vi "ROS_MasterSaveHTML.vi"(3 "Latest Request":string, 5 "Current":T3) -> ()   [LabVIEW 2015]
doc: "saves HTML file for Master"
uses:
  ROS_Master.ctl
  ROS_Topic.ctl
  ROS_Node.ctl
  ROS_Service.ctl
  SubVIs/_ROSControl.ctl
  SubVIs/_ROSDirection.ctl
panel:
  in  "ROS":T1={"topic port"=0, "Node"="", "topic"="", "type"="", "node port"=0, "error "={"status"=FALSE, "code"=0, "source"=""}, "Direction"=enum."Node", "Update (ms)"=1, "FIFO size"=1}
  out "HTML":string
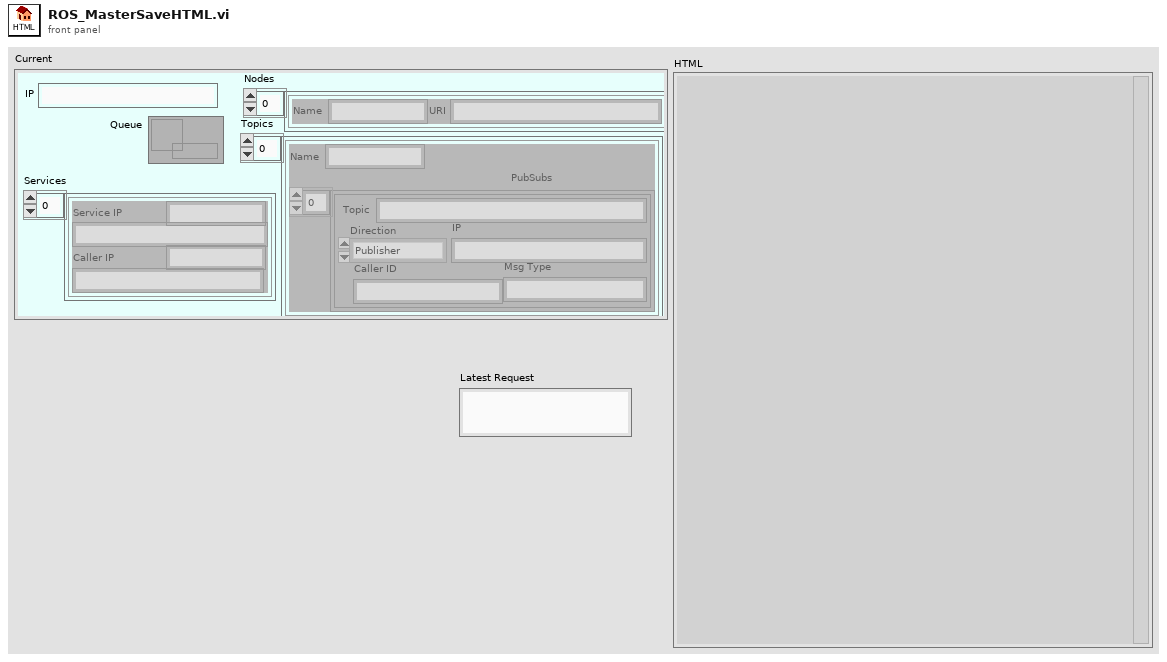
[diagram p1: front panel]
types:
  T1 = typedef "_ROSControl.ctl" = cluster{"topic port":u16, "Node":string, "topic":string, "type":string, "node port":u16, "error ":errorcluster, "Direction":T2, "Update (ms)":u16, "FIFO size":u16}
  T2 = typedef "_ROSDirection.ctl" = enum16{"Node", "Publisher", "Subscriber", "ServiceClient", "ServiceProvider"}
  T3 = typedef "ROS_Master.ctl" = cluster{"IP":string, "Topics":cluster{"Name":string, "PubSubs":T4[]}[], "Nodes":T5[], "Services":T6[], "Queue":refnum<queue>}
  T4 = typedef "ROS_Topic.ctl" = cluster{"Caller ID":string, "IP":string, "Msg Type":string, "Direction":enum16{"Publisher", "Subscriber"}, "Topic":string}
  T5 = typedef "ROS_Node.ctl" = cluster{"Name":string, "URI":string}
  T6 = typedef "ROS_Service.ctl" = cluster{"Service":string, "Service IP":string, "Caller IP":string, "Caller ID":string}
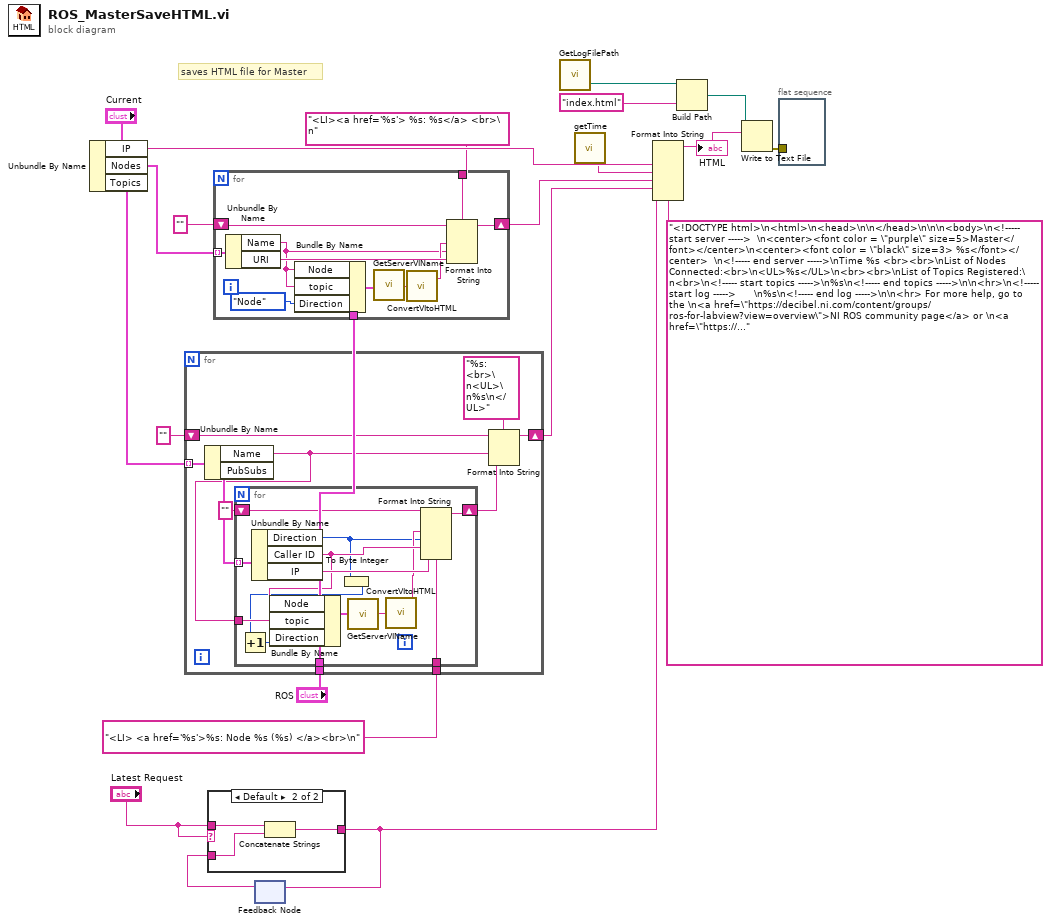
[diagram p0: block diagram]
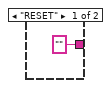
[diagram p2: hidden frame]
diagram:
  # "saves HTML file for Master"
  n1 = Unbundle By Name("Current") -> ("IP"=w19:string, "Nodes"=w18:T5[], "Topics"=w14:cluster{"Name":string, "PubSubs":T4[]}[])
  n2 = for {
    tunnel: w14 -> [w31] mode=indexing
    shift-right: [w29] -> w13
    shift-left: "" -> [w28]
    tunnel: "ROS" -> [w24]
    tunnel: "<LI> <a href='%s'>%s: Node %s (%s) </a><br>\n" ("format string") -> [w23]
    n3 = Unbundle By Name(w31) -> ("Name"=w22:string, "PubSubs"=w27:T4[])
    n4 = for {
      tunnel: w27 -> [w45] mode=indexing
      shift-right: [w42] -> w25
      shift-left: "" -> [w43]
      tunnel: w24 -> [w39]
      tunnel: w22 -> [w37]
      tunnel: w23 -> [w36]
      n5 = Unbundle By Name(w45) -> ("Direction"=w34:enum16{"Publisher", "Subscriber"}, "Caller ID"=w38:string, "IP"=w44:string)
      n6 = To Byte Integer(number=w34) -> (8bit integer=w32:i8)
      n7 = Increment(x=w32) -> (x+1=w33:i8)
      n8 = Bundle By Name(cluster=w39, "Node"=w38, "topic"=w37, "Direction"=w33) -> (w40:T1)
      n9 = call "GetServerVIName.vi"("ROS"=w40) -> ("vi name"=w41:string)
      n10 = call "ConvertVItoHTML.vi"("vi name"=w41) -> ("Htm log name"=w35:string)  [unwired: 1 out]
      n11 = Format Into String(format string=w36, initial string=w43, w35, w34, w38, w44) -> (resulting string=w42:string)  [unwired: 1 in, 1 out]
    }
    n12 = Format Into String(format string="%s: <br>\n<UL>\n%s\n</UL>", initial string=w28, w22, w25) -> (resulting string=w29:string)  [unwired: 1 in, 1 out]
  }
  n13 = for {
    tunnel: w18 -> [w56] mode=indexing
    shift-right: [w55] -> w16
    shift-left: "" -> [w54]
    tunnel: "<LI><a href='%s'> %s: %s</a> <br>\n" ("format string") -> [w53]
    tunnel: "ROS" -> [w51]
    n14 = Unbundle By Name(w56) -> ("Name"=w47:string, "URI"=w52:string)
    n15 = Bundle By Name(cluster=w51, "Node"=w47, "topic"=w47, "Direction"=_ROSDirection."Node") -> (w50:T1)
    n16 = call "GetServerVIName.vi"("ROS"=w50) -> ("vi name"=w49:string)
    n17 = call "ConvertVItoHTML.vi"("vi name"=w49) -> ("Htm log name"=w48:string)  [unwired: 1 out]
    n18 = Format Into String(format string=w53, initial string=w54, w48, w47, w52) -> (resulting string=w55:string)  [unwired: 1 in, 1 out]
  }
  n19 = feedback #1() -> (w1:string)  [unwired: 1 in]
  n20 = case shown="Default" "Latest Request" {
    tunnel: "Latest Request" -> [_ w60]
    tunnel: ["" w59] -> w2
    tunnel: w1 -> [_ w58]
    frame "RESET" {
    }
    frame Default {
      n21 = Concatenate Strings(w60, w58) -> (w59:string)
    }
  }
  n22 = feedback-in #1(w2) -> ()
  n23 = call "GetLogFilePath.vi"() -> ("LogFolder"=w11:path)  [unwired: 2 in, 1 out]
  n24 = call "getTime.vi"() -> ("Current Time"=w4:string)  [unwired: 1 in]
  n25 = Format Into String(format string="<!DOCTYPE html>\n<html>\n<head>\n\n</head>\n\n\n<body>\n<!----- start server ----->  \n<center><font color = \"purple\" size=5>Master</font></center>\n<center><font color = \"black\" size=3> %s</font></center>  \n<!----- end server ----->\nTime %s <br><br>\nList of Nodes Connected:<br>\n<UL>%s</UL>\n<br><br>\nList of Topics Registered:\n<br>\n<!----- start topics ----->\n%s\n<!----- end topics ----->\n\n<hr>\n<!----- start log ----->      \n%s\n<!----- end log ----->\n\n<hr> For more help, go to the \n<a href=\"https://decibel.ni.com/content/groups/ros-for-labview?view=overview\">NI ROS community page</a> or \n<a href=\"https://github.com/tuftsBaxter/ROS-for-LabVIEW-Software\">the LVROS Github</a>\n</body>\n</html>" ("regular expression"), w19, w4, w16, w13, w2) -> (resulting string=w12:string)  [unwired: 2 in, 1 out]
  "HTML" <- w12
  n26 = Build Path(base path=w11, name or relative path="index.html" ("Server name")) -> (appended path=w9:path)
  n27 = Write to Text File(file (use dialog)=w9, text=w12) -> (error out=w5:errorcluster)  [unwired: 2 in, 2 out]
  n28 = flat-sequence {
    tunnel: w5 -> [_]
    frame #0 {
    }
  }
